vi "Write and Read Multiple Holding Registers.vi"(4 "read count":u16, 6 "read operation starting address":u16, 8 "error in (no error)":errorcluster, 9 "values to write":u16[](array[numeric]), 10 "write operation starting address":u16, 11 "MB CR in":refnum<class "Modbus Master CR API.lvclass">) -> (0 "error out":errorcluster, 1 "values read":u16[](array[numeric]), 3 "MB CR out":refnum<class "Modbus Master CR API.lvclass">)   [LabVIEW 2021, in "Modbus Master CR API.lvclass"]
doc: "Writes and reads values to and from contiguous holding registers."
uses:
  Modbus Master CR API.lvclass
  D:/my_projects/projects/Algorithms/Labview/21/Modbus_v121c/API/Modbus API.lvclass
  Modbus API.lvclass/Modbus API.ctl
  Network Protocol/MB/Modbus Master CR.lvclass/Modbus Master CR.ctl
  Read Network Protocol.vi
  Network Protocol/MB/Modbus Master CR.lvclass
  Data Model/Device Data Model.lvclass
  Modbus Master CR API.lvclass/Modbus Master CR API.ctl
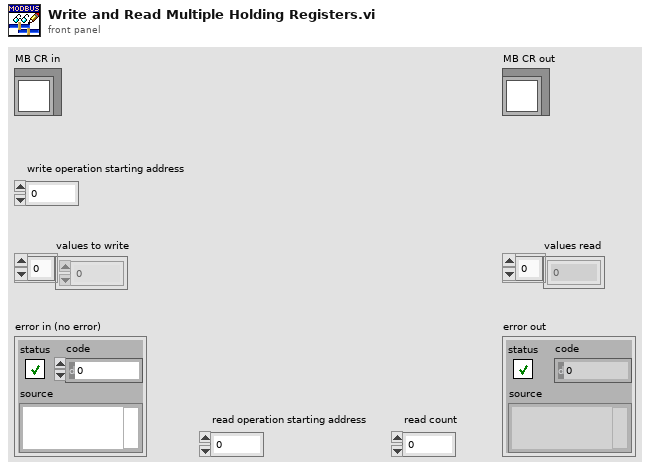
[diagram p1: front panel]
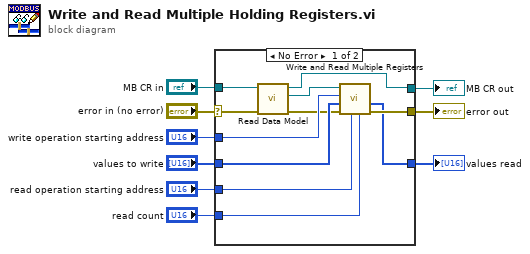
[diagram p0: block diagram]
diagram:
  n1 = case shown="No Error" "error in (no error)" {
    selector: "error in (no error)" -> [w14 w22]
    tunnel: [w20 w22] -> w1
    tunnel: "MB CR in" -> [w10 w21]
    tunnel: [w11 w21] -> w8
    tunnel: [w19 _] -> w7
    tunnel: "read operation starting address" -> [w18 _]
    tunnel: "read count" -> [w17 _]
    tunnel: "write operation starting address" -> [w16 _]
    tunnel: "values to write" -> [w15 _]
    frame No Error {
      n2 = call "Read Data Model.vi"("error in (no error)"=w14, "MB CR in"=w10) -> ("error out"=w13:errorcluster, "device data model"=w12:refnum<class "Device Data Model.lvclass">, "MB CR out"=w11:refnum<class "Modbus Master CR API.lvclass">)  [unwired: 7 in]
      n3 = call-dynamic "Write and Read Multiple Registers.vi"("read count"=w17, "read starting address"=w18, "error in"=w13, "write values"=w15, "write starting address"=w16, "device data model in"=w12) -> ("error out"=w20:errorcluster, "read values"=w19:u16[])  [unwired: 3 in, 1 out]
    }
    frame Error {
    }
  }
  "error out" <- w1
  "MB CR out" <- w8
  "values read" <- w7
